vi "Close.vi"(8 "error in (no error)":errorcluster, 11 "EPOS4 Settings In":T1={"VISA resource name"="", "axis"={"keyHandle"=0, "nodeId"=1}, "Simulated?"=FALSE}) -> (0 "error out":errorcluster, 1 "Connection Error":bool, 3 "EPOS4 Settings Out":T1={"VISA resource name"="", "axis"={"keyHandle"=0, "nodeId"=1}, "Simulated?"=FALSE})   [LabVIEW 2018, in "EPOS4.lvlib"]
uses:
  EPOS4.lvlib
  Controls/EPOS Communication Settings.ctl
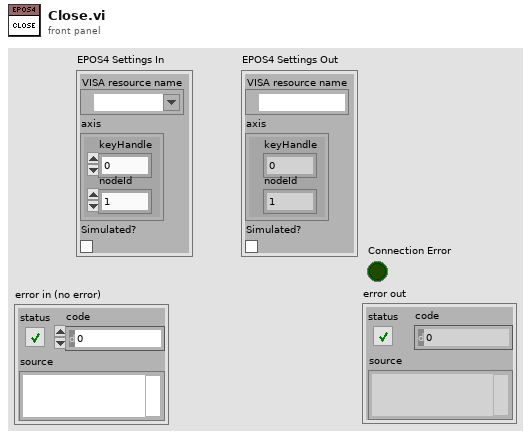
[diagram p1: front panel]
types:
  T1 = typedef "EPOS4.lvlib/EPOS Communication Settings.ctl" = cluster{"VISA resource name":refnum<visa-resource-name>, "axis":cluster{"keyHandle":u32, "nodeId":u16}, "Simulated?":bool}
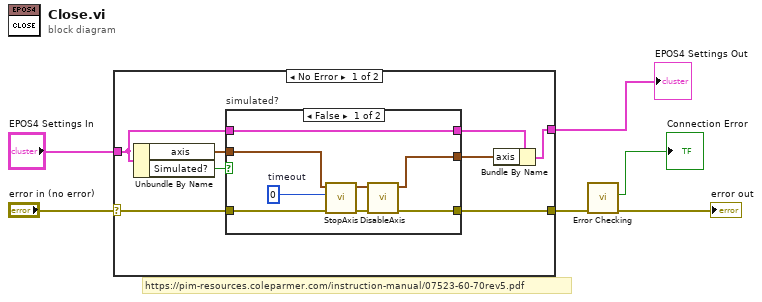
[diagram p0: block diagram]
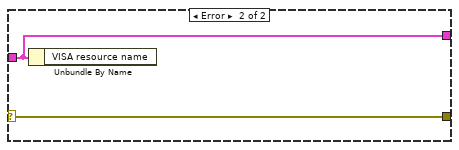
[diagram p3: hidden frame]
diagram:
  # "https://pim-resources.coleparmer.com/instruction-manual/07523-60-70rev5.pdf"
  n1 = case shown="No Error" "error in (no error)" {
    selector: "error in (no error)" -> [w12 w27]
    tunnel: [w9 w27] -> w4
    tunnel: [w13 w26] -> w1
    tunnel: "EPOS4 Settings In" -> [w10 w26]
    frame No Error {
      n2 = Unbundle By Name(w10) -> ("axis"=w11:cluster{"keyHandle":u32, "nodeId":u16}, "Simulated?"=w14:bool)
      n3 = case "simulated?" shown="False" w14 {
        tunnel: w12 -> [w19 w23]
        tunnel: w11 -> [w21 w24]
        tunnel: w10 -> [w20 w25]
        tunnel: [w15 w23] -> w9
        tunnel: [w17 w24] -> w8
        tunnel: [w20 w25] -> w7
        frame False {
          w22 = u32 0  # timeout
          n4 = call "StopAxis.vi"("error in (no error)"=w19, "timeout"=w22, "axis in"=w21) -> ("error out"=w16:errorcluster, "axis out"=w18:cluster{"keyHandle":u32, "nodeId":u16})  [unwired: 3 in]
          n5 = call "DisableAxis.vi"("error in (no error)"=w16, "axis in"=w18) -> ("error out"=w15:errorcluster, "axis out"=w17:cluster{"keyHandle":u32, "nodeId":u16})  [unwired: 4 in]
        }
        frame True {
        }
      }
      n6 = Bundle By Name(cluster=w7, "axis"=w8) -> (w13:T1)
    }
    frame Error {
      n7 = Unbundle By Name(w26) -> ()  [unwired: 1 out]
    }
  }
  "EPOS4 Settings Out" <- w1
  n8 = call "Error Checking.vi"("error in (no error)"=w4) -> ("error out"=→"error out":errorcluster, "Connection Error"=→"Connection Error":bool)  [unwired: 8 in, 1 out]
